vi "ex8-5.vi"   [LabVIEW 2009]
uses:
  <vilib>/NXT/Dual Mode Library/Waits/Wait_Num.vi
  <vilib>/NXT/Dual Mode Library/Display/drawPicture.vi
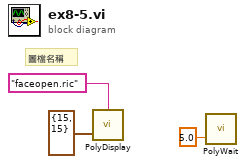
[diagram p0: block diagram]
diagram:
  # "圖檔名稱"
  n1 = call-poly <vilib>:"PolyDisplay.vi"("Origin"=cluster{"X":i16, "Y":i16} {"X"=15, "Y"=15}, "Filename (*.ric)"="faceopen.ric") -> ()  [unwired: 2 in, 1 out]
  n2 = call-poly <vilib>:"PolyWait.vi"("Time (1 sec)"=sgl 5.0) -> ()  [unwired: 3 in, 1 out]
